vi "Center Finder Corelation.vi"(4 "Xmin":u32, 5 "Xmax":u32, 6 "Y_positions":i16[](array[numeric])=[0, 0, 0, 0, 0, 0, 0, 0, 0, 1, 1, 1, 1, 1, 1, 1, 1, 1, 1, 1, 1, 1, 1, 1, 1, 1, 1, 1, 1, 1, 1, 1, 1, 1, 1, 1, 1, 1, 1, 1, 1, 1, 0, 0, 0, 0, 0, 0, 0, 0, 0, 0, 0, 0, 0, 0, 0, 0, 0, 0, 0, 0, 0, 0, 0, 0, 0, 0, 0, 0, 0, 0, 0, 0, 0, 0, 0, 0, 0, 0, 0, 0, 0, 0, 0, 0, 0, 0, 0, 0, 0, 0, 0, 0, 0, 0, 0, 0, 0, 0], 7 "Ymax":u32, 8 "X_positions":i16[](array[numeric])=[1, 1, 1, 1, 1, 1, 1, 1, 1, 1, 1, 1, 1, 1, 1, 1, 1, 0, 0, 0, 0, 0, 0, 0, 0, 0, 0, 0, 0, 0, 0, 0, 0, 0, 0, 0, 0, 0, 0, 0, 0, 0, 0, 0, 0, 0, 0, 0, 0, 0, 0, 0, 0, 0, 0, 0, 0, 0, 0, 0, 0, 0, 0, 0, 0, 0, 0, 0, 0, 0, 0, 0, 0, 0, 0, 0, 0, 0, 0, 0, 0, 0, 0, 1, 1, 1, 1, 1, 1, 1, 1, 1, 1, 1, 1, 1, 1, 1, 1, 1], 9 "Picture":u8[][](array[numeric]), 11 "Ymin":u32) -> (0 "X":u32, 1 "Y":u32, 3 "Grade":u32)   [LabVIEW 2015]
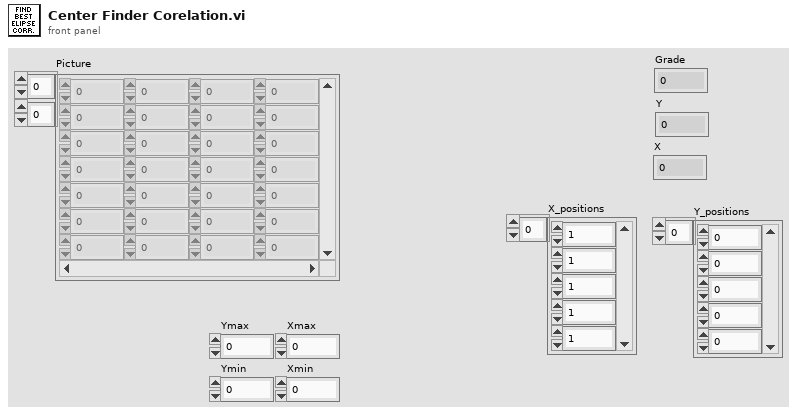
[diagram p1: front panel]
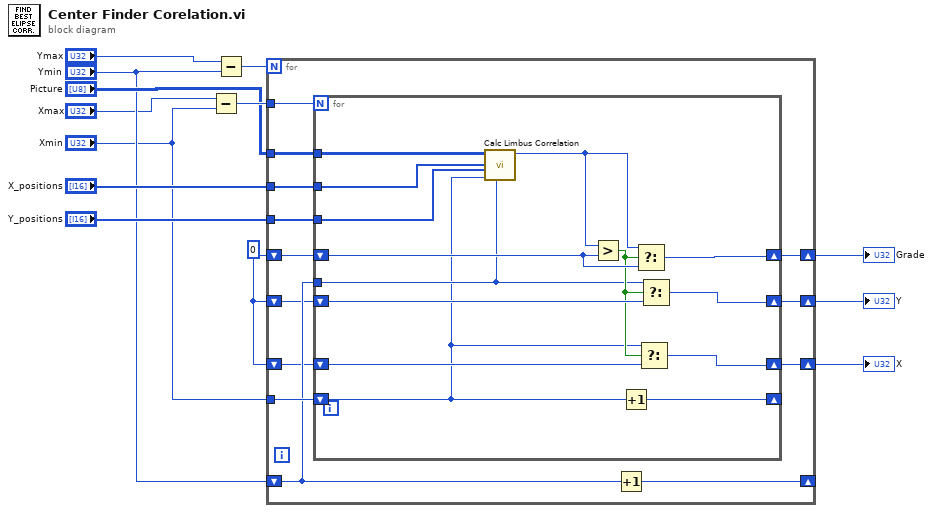
[diagram p0: block diagram]
diagram:
  w9 = u32 0 ("Grade")
  n1 = Subtract(x="Xmax", y="Xmin") -> (x-y=w13:u32)
  n2 = Subtract(x="Ymax", y="Ymin") -> (x-y=w8:u32)
  n3 = for {
    N: w8 -> [_]
    tunnel: "Picture" -> [w26]
    tunnel: w13 -> [w25]
    tunnel: "Xmin" -> [w24]
    shift-right: [w23] -> _
    shift-left: "Ymin" -> [w22]
    shift-right: [w20] -> w12
    shift-left: w9 -> [w21]
    shift-right: [w19] -> w11
    shift-left: w9 -> [w17]
    shift-right: [w18] -> w10
    shift-left: w9 -> [w16]
    tunnel: "X_positions" -> [w15]
    tunnel: "Y_positions" -> [w14]
    n4 = for {
      N: w25 -> [_]
      tunnel: w26 -> [w32]
      shift-right: [w40] -> _
      shift-left: w24 -> [w27]
      tunnel: w22 -> [w31]
      shift-right: [w38] -> w20
      shift-left: w21 -> [w39]
      shift-right: [w37] -> w19
      shift-left: w17 -> [w35]
      shift-right: [w36] -> w18
      shift-left: w16 -> [w34]
      tunnel: w15 -> [w29]
      tunnel: w14 -> [w28]
      n5 = call "Calc Limbus Correlation.vi"("Y"=w31, "X"=w27, "Y_positions"=w28, "X_positions"=w29, "Picture"=w32) -> ("Grade"=w30:u32)  [unwired: 6 in]
      n6 = Greater?(x=w30, y=w39) -> (0:w33:bool)
      n7 = Increment(x=w27) -> (x+1=w40:u32)
      n8 = Select(t=w30, s=w33, f=w39) -> (s? t:f=w38:u32)
      n9 = Select(t=w27, s=w33, f=w34) -> (s? t:f=w36:u32)
      n10 = Select(t=w31, s=w33, f=w35) -> (s? t:f=w37:u32)
    }
    n11 = Increment(x=w22) -> (x+1=w23:u32)
  }
  "Grade" <- w12
  "Y" <- w11
  "X" <- w10
